vi "Starting.vi"(4 "Queue of Async Elements":refnum<queue>, 7 "Actor in":refnum<class "Actor.lvclass">, 9 "Attributes":refnum<class "Attributes.lvclass">, 10 "Refs":refnum<class "Refs.lvclass">) -> (0 "Error out":errorcluster, 5 "Actor out":refnum<class "Actor.lvclass">)   [LabVIEW 2025, in "jettl.lvlib" / "Event Transport.lvlib"]
uses:
  Event Transport.lvlib
  Actor/Actor.lvclass
  Attributes/Attributes.lvclass
  Refs/Refs.lvclass
  Async Elements.ctl
  jettl.lvlib
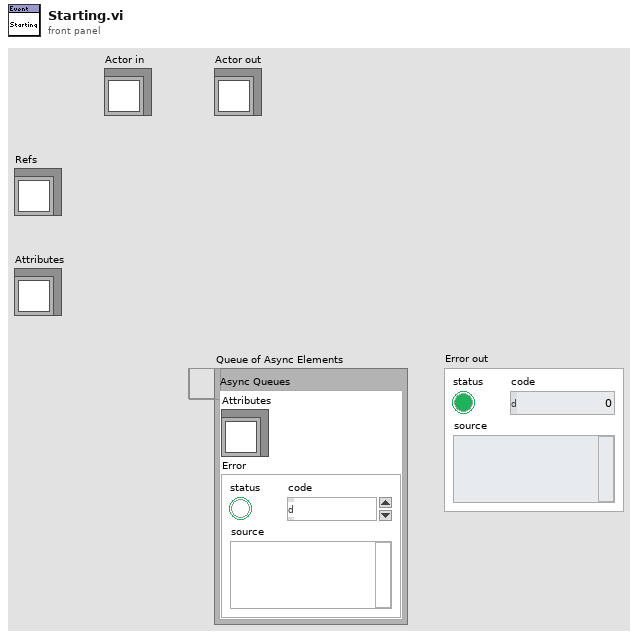
[diagram p1: front panel]
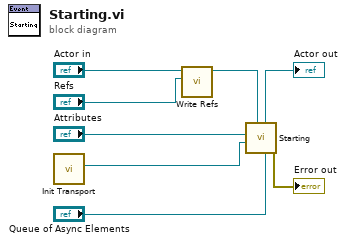
[diagram p0: block diagram]
diagram:
  n1 = call "Init Transport.vi"() -> ("Transport"=w7:refnum<class "Transport.lvclass">)  [unwired: 11 in]
  n2 = call-dynamic "Write Refs.vi"("Refs"="Refs", "Actor in"="Actor in") -> ("Actor out"=w3:refnum<class "Actor.lvclass">)  [unwired: 9 in]
  n3 = call "Starting.vi"("Queue of Async Elements"="Queue of Async Elements", "Actor in"=w3, "Transport"=w7, "Attributes"="Attributes") -> ("Error out"=→"Error out":errorcluster, "Actor out"=→"Actor out":refnum<class "Actor.lvclass">)  [unwired: 6 in]
